vi "Update Device.vi"(8 "error in (no error)":errorcluster, 10 "Device":refnum<class "Device.lvclass">, 11 "HAL Manager in":refnum<class "HAL Manager.lvclass">) -> (0 "error out":errorcluster, 3 "HAL Manager out":refnum<class "HAL Manager.lvclass">)   [LabVIEW 2020, in "HAL.lvlib" / "HAL Manager.lvclass"]
uses:
  HAL Manager.lvclass
  Device/Device.lvclass
  HAL Manager.lvclass/HAL Manager.ctl
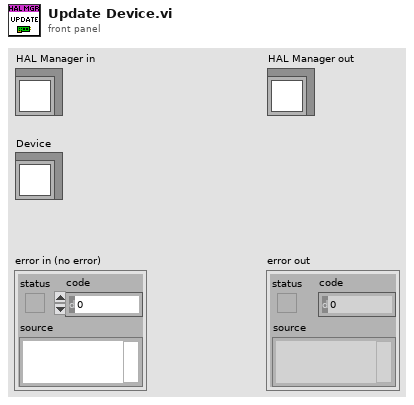
[diagram p1: front panel]
types:
  T1 = typedef "HAL.lvlib/HAL Manager.lvclass/Ref Data.ctl" = cluster{"Devices":refnum<class "Device.lvclass">[], "Type":string[], "Models":string[], "Name":string[]}
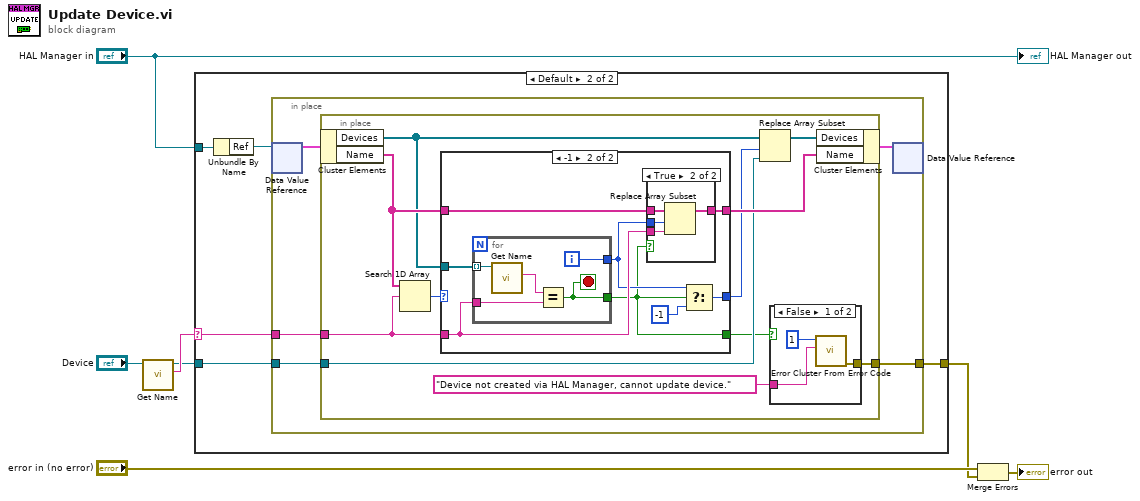
[diagram p0: block diagram]
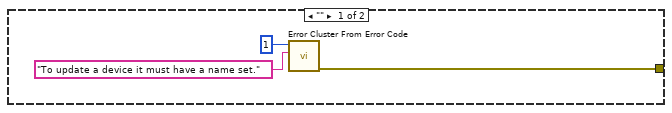
[diagram p2: hidden frame]
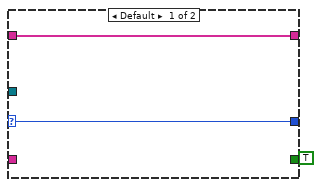
[diagram p4: hidden frame]
diagram:
  n1 = call "Get Name.vi"("Device in"="Device") -> ("Name"=w5:string, "Device out"=w4:refnum<class "Device.lvclass">)  [unwired: 8 in, 1 out]
  n2 = case shown="Default" w5 {
    selector: w5 -> [_ w13]
    tunnel: "HAL Manager in" -> [_ w14]
    tunnel: w4 -> [_ w12]
    tunnel: [w8 w11] -> w1
    frame "" {
      n3 = call <vilib>:"Error Cluster From Error Code.vi"("error message (\"\")"="To update a device it must have a name set.", "error code (0)"=1) -> ("error out"=w8:errorcluster)  [unwired: 7 in]
    }
    frame Default {
      n4 = Unbundle By Name(w14) -> ("Ref"=w15:refnum<data-value>)
      n5 = in-place {
        in-place-border: w13 -> [w19]
        in-place-border: w12 -> [w17]
        in-place-border: [w16] -> w11
        n6 = in-place-dvr #1(w15) -> (w20:T1)  [unwired: 1 out]
        n7 = in-place {
          in-place-border: w19 -> [w30]
          in-place-border: w17 -> [w24]
          in-place-border: [w21] -> w16
          n8 = in-place-cluster #2(w20) -> ("Devices"=w27:refnum<class "Device.lvclass">[], "Name"=w29:string[])
          n9 = Search 1D Array(1D array=w29, element=w30) -> (index of element=w31:i32)  [unwired: 1 in]
          n10 = case shown="-1" w31 {
            selector: w31 -> [w35 _]
            tunnel: w30 -> [_ w43]
            tunnel: w29 -> [w36 w44]
            tunnel: [w36 w42] -> w28
            tunnel: [w35 w40] -> w25
            tunnel: w27 -> [_ w38]
            tunnel: [_ w37] -> w23
            frame Default {
              (unwired) TRUE
            }
            frame -1 {
              n11 = for {
                tunnel: w43 -> [w54]
                tunnel: [w52] -> w37
                tunnel: [w51] -> w41
                tunnel: w38 -> [w50] mode=indexing
                i -> [w51]
                stop <- w52 stop-if-true
                n12 = call "Get Name.vi"("Device in"=w50) -> ("Name"=w53:string)  [unwired: 8 in, 2 out]
                n13 = Equal?(x=w53, y=w54) -> (x = y?=w52:bool)
              }
              n14 = case shown="True" w37 {
                tunnel: w44 -> [w45 w49]
                tunnel: w43 -> [_ w48]
                tunnel: w41 -> [_ w47]
                tunnel: [w45 w46] -> w42
                frame False {
                }
                frame True {
                  n15 = Replace Array Subset(array=w49, new element=w48, index=w47) -> (w46:string[])
                }
              }
              n16 = Select(t=w41, s=w37, f=-1) -> (s? t:f=w40:i32)
            }
          }
          n17 = Replace Array Subset(array=w27, new element=w24, index=w25) -> (w26:refnum<class "Device.lvclass">[])
          n18 = case shown="False" w23 {
            tunnel: "Device not created via HAL Manager, cannot update device." -> [w34 _]
            tunnel: [w32 _] -> w21
            frame False {
              n19 = call <vilib>:"Error Cluster From Error Code.vi"("error message (\"\")"=w34, "error code (0)"=1) -> ("error out"=w32:errorcluster)  [unwired: 7 in]
            }
            frame True {
            }
          }
          n20 = in-place-cluster #2("Devices"=w26, "Name"=w28) -> (w18:T1)
        }
        n21 = in-place-dvr #1(w18) -> ()  [unwired: 2 out]
      }
    }
  }
  n22 = Merge Errors("error in (no error)", w1) -> (→"error out":errorcluster)
  "HAL Manager out" <- "HAL Manager in"
